vi "Update Device emperature.vi"(8 "error in (no error)":errorcluster, 10 "Data Cluster":T1, 11 "Message Queue in":refnum<class "Delacor_lib_QMH_Message Queue.lvclass">) -> (0 "error out":errorcluster, 2 "Data Cluster out":T1)   [LabVIEW 2015, in "Tool Module.lvlib"]
uses:
  Tool Module.lvlib
  Module Data--cluster.ctl
  Event Logger Library/Event Log/EventLog.lvclass
  _STATUS Typedef--cluster.ctl
  Timer State Return Typedef.ctl
  Get All Inspect Data (Reply Payload)--cluster.ctl
  _Sample Data Rtn Cluster--typedef.ctl
  _Inspection Limits cluster--typedef.ctl
  <vilib>/Delacor/Delacor QMH/Libraries/Message Queue_class/Delacor_lib_QMH_Message Queue.lvclass
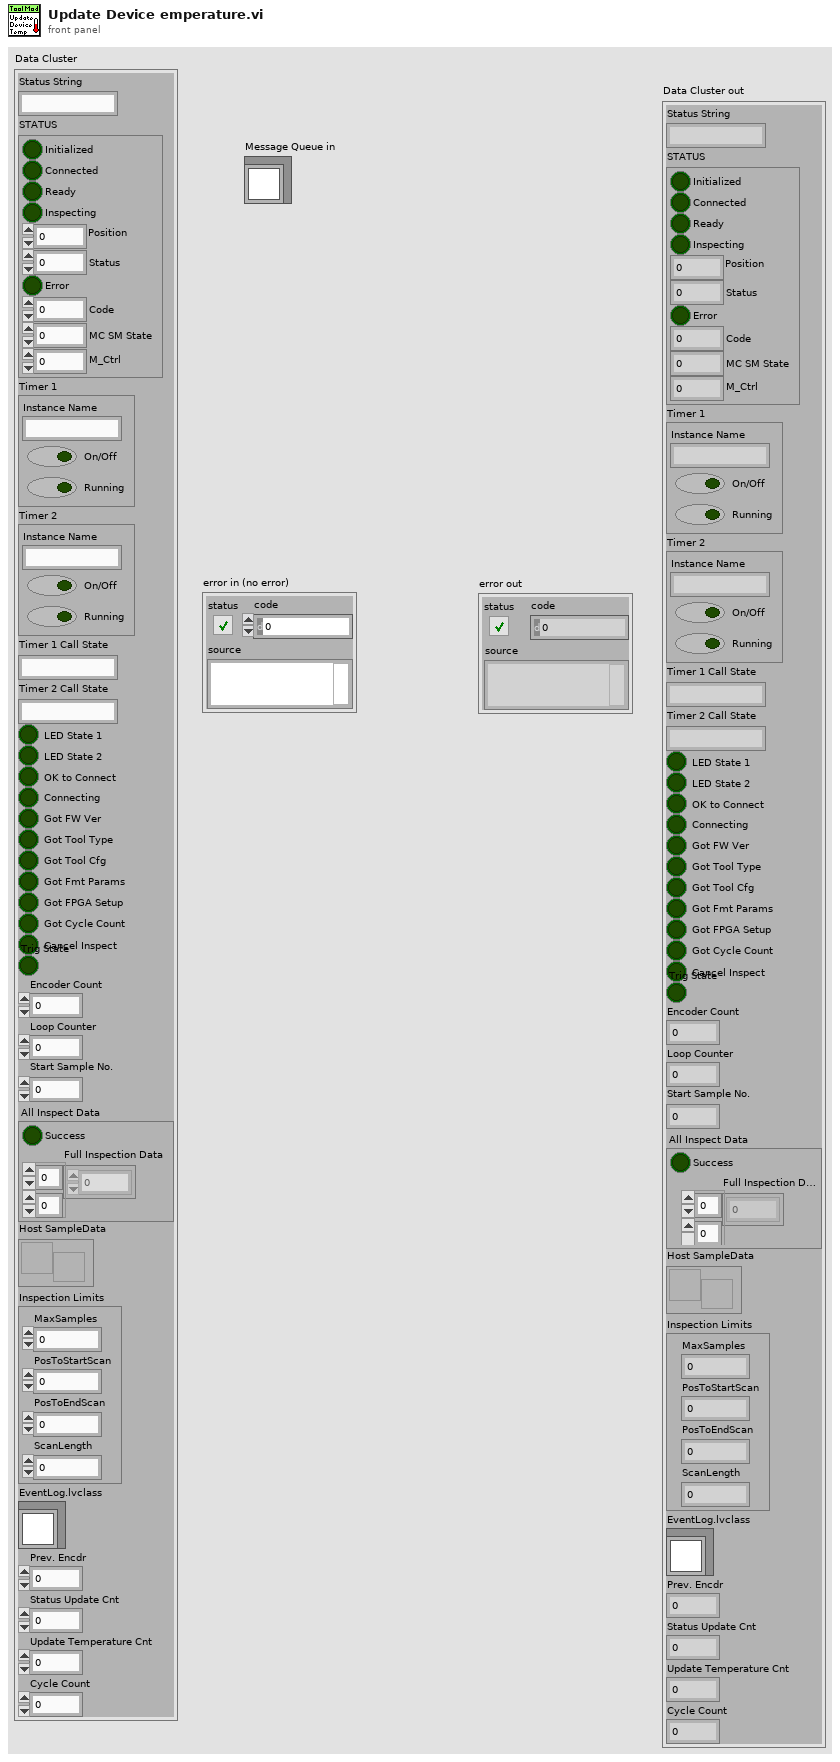
[diagram p1: front panel]
types:
  T1 = typedef "Tool Module.lvlib/Module Data--cluster.ctl" = cluster{"Status String":string, "STATUS":T2, "Timer 1":T3, "Timer 2":T3, "Timer 1 Call State":string, "Timer 2 Call State":string, "LED State 1":bool, "LED State 2":bool, "OK to Connect":bool, "Connecting":bool, "Got FW Ver":bool, "Got Tool Type":bool, "Got Tool Cfg":bool, "Got Fmt Params":bool, "Got FPGA Setup":bool, "Got Cycle Count":bool, "Cancel Inspect":bool, "Trig State":bool, "Encoder Count":i32, "Loop Counter":i32, "Start Sample No.":u32, "All Inspect Data ":T4, "Host SampleData":refnum<notifier>, "Inspection Limits":T5, "EventLog.lvclass":refnum<class "EventLog.lvclass">, "Prev. Encdr":i32, "Status Update Cnt":i32, "Update Temperature Cnt":i32, "Cycle Count":i32}
  T2 = typedef "Tool Module.lvlib/_STATUS Typedef--cluster.ctl" = cluster{"Initialized":bool, "Connected":bool, "Ready":bool, "Inspecting":bool, "Position":dbl, "Status":u16, "Error":bool, "Code":i32, "MC SM State":u16, "M_Ctrl":u16}
  T3 = typedef "Tool Module.lvlib/Timer State Return Typedef.ctl" = cluster{"Instance Name":string, "On/Off":bool, "Running":bool}
  T4 = typedef "Tool Module.lvlib/Get All Inspect Data (Reply Payload)--cluster.ctl" = cluster{"Success":bool, "Full Inspection Data":u32[][]}
  T5 = typedef "Tool Module.lvlib/_Inspection Limits cluster--typedef.ctl" = cluster{"MaxSamples":i32, "PosToStartScan":i32, "PosToEndScan":i32, "ScanLength":i32}
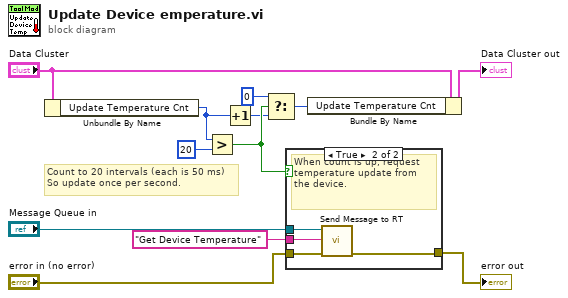
[diagram p0: block diagram]
diagram:
  # "Count to 20 intervals (each is 50 ms)\nSo update once per second."
  n1 = Unbundle By Name("Data Cluster") -> ("Update Temperature Cnt"=w5:i32)
  n2 = Greater?(x=w5, y=20) -> (0:w3:bool)
  n3 = Increment(x=w5) -> (x+1=w1:i32)
  n4 = Select(t=0, s=w3, f=w1) -> (s? t:f=w4:i32)
  n5 = case shown="True" w3 {
    tunnel: "Message Queue in" -> [_ w17]
    tunnel: "error in (no error)" -> [w13 w16]
    tunnel: "Get Device Temperature" ("Message") -> [_ w15]
    tunnel: [w13 w14] -> w2
    frame False {
    }
    frame True {
      # "When count is up, request temperature update from the device."
      n6 = call "Send Message to RT.vi"("error in (no error)"=w16, "Message"=w15, "Message Queue in"=w17) -> ("error out"=w14:errorcluster)  [unwired: 7 in, 1 out]
    }
  }
  "error out" <- w2
  n7 = Bundle By Name(cluster="Data Cluster", "Update Temperature Cnt"=w4) -> (→"Data Cluster out":T1)
